vi "Start Serving.vi"(8 "error in (no error)":errorcluster, 11 "DIMActor in":refnum<class "DIMActor.lvclass">) -> (0 "error out":errorcluster, 3 "DIMActor out":refnum<class "DIMActor.lvclass">)   [LabVIEW 2012, in "DIMActor.lvlib" / "DIMActor.lvclass"]
doc: "Start serving."
uses:
  DIMActor.lvclass
  DIMActor.lvclass/DIMActor.ctl
  SVN/LV2009/GPL/lib.lib/DimLVEvent/LVDimInterface/LVDimInterface.lvlib
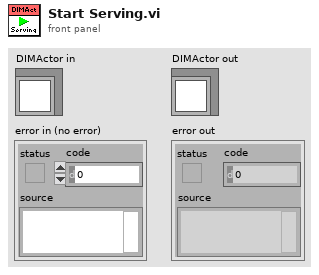
[diagram p1: front panel]
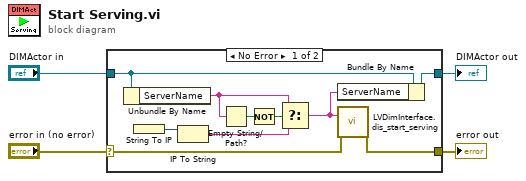
[diagram p0: block diagram]
diagram:
  n1 = case shown="No Error" "error in (no error)" {
    selector: "error in (no error)" -> [w6 w16]
    tunnel: [w5 w16] -> w3
    tunnel: [w7 w15] -> w1
    tunnel: "DIMActor in" -> [w8 w15]
    frame No Error {
      n2 = Unbundle By Name(w8) -> ("ServerName"=w10:string)
      n3 = String To IP() -> (0:w14:u32)  [unwired: 1 in]
      n4 = IP To String(2:w14) -> (0:w11:string)  [unwired: 1 in]
      n5 = Empty String/Path?(string/path=w10) -> (empty?=w13:bool)
      n6 = Not(x=w13) -> (.not. x?=w12:bool)
      n7 = Select(t=w10, s=w12, f=w11) -> (s? t:f=w9:string)
      n8 = Bundle By Name(cluster=w8, "ServerName"=w9) -> (w7:refnum<class "DIMActor.lvclass">)
      n9 = call "LVDimInterface.dis_start_serving.vi"("serverName"=w9, "error in (no error)"=w6) -> ("error out"=w5:errorcluster)  [unwired: 16 in, 1 out]
    }
    frame Error {
    }
  }
  "error out" <- w3
  "DIMActor out" <- w1
